vi "Add lvlib To Project.vi"(6 "Created Library File Path":path, 8 "error in":errorcluster, 9 "Template Library File Path":path, 10 "Target":refnum<vi>) -> (0 "error out":errorcluster)   [LabVIEW 2020, in "_Template.lvlib" / "_Template.lvclass"]
uses:
  _Template.lvclass
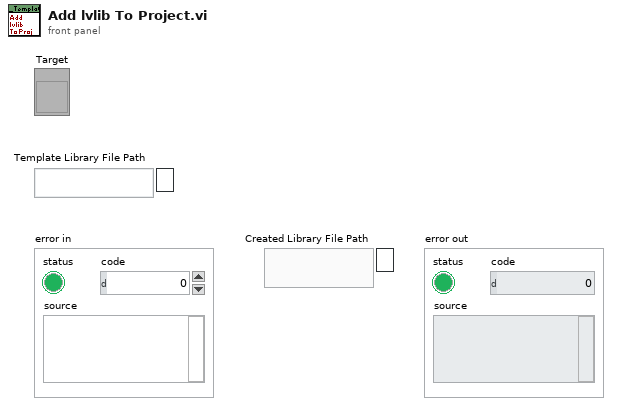
[diagram p1: front panel]
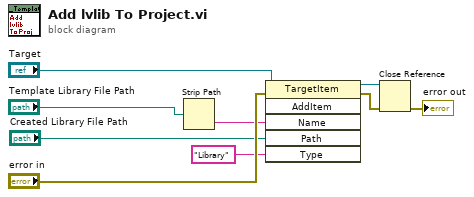
[diagram p0: block diagram]
diagram:
  n1 = Strip Path(path="Template Library File Path") -> (name=w3:string)  [unwired: 1 out]
  n2 = invoke class="TargetItem" method="AddItem"(reference="Target", error in="error in", "Name"=w3, "Path"="Created Library File Path", "Type"="Library") -> (reference out=w7:refnum<vi>, error out=w6:errorcluster)  [unwired: 1 in, 4 out]
  n3 = Close Reference(reference=w7, error in (no error)=w6) -> (error out=→"error out":errorcluster)
